vi "execute_value_write_policy.vi"(8 "error in (no error)":errorcluster, 9 "Publish Time":timestamp, 10 "New Topic Value":variant, 11 "BasicSubscription In":refnum<class "BasicSubscription.lvclass">) -> (0 "error out":errorcluster, 3 "BasicSubscription Out":refnum<class "BasicSubscription.lvclass">)   [LabVIEW 2015, in "SubscriptionPolicy.lvlib" / "BasicSubscription.lvclass"]
uses:
  BasicSubscription.lvclass
  IMediator/ISubscriptionPolicy/ISubscriptionPolicy.lvclass/ISubscriptionPolicy.ctl
  IMediator/ITransport/ITransport.lvclass
  IMediator/ISubscriptionPolicy/ISubscriptionPolicy.lvclass
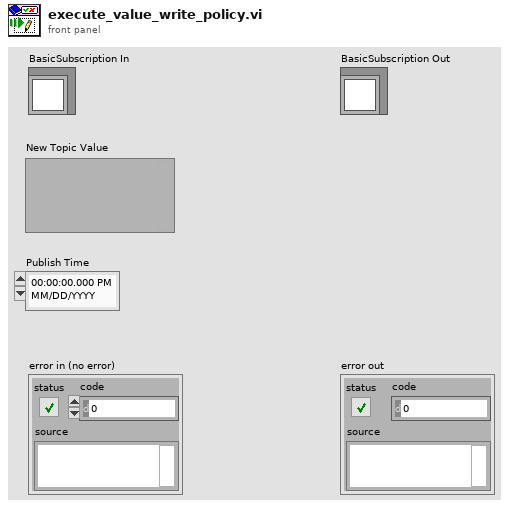
[diagram p1: front panel]
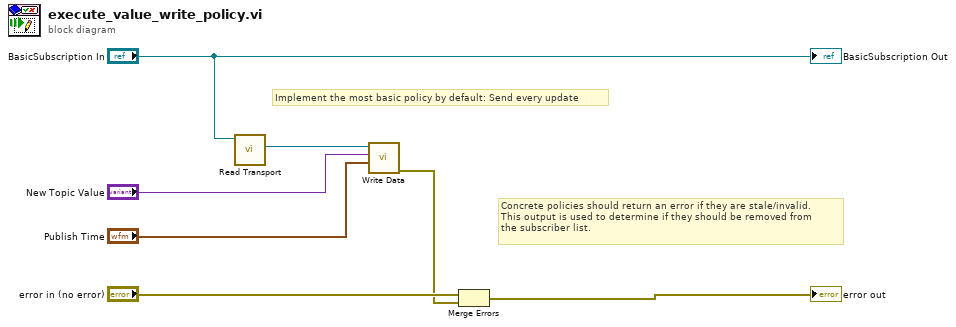
[diagram p0: block diagram]
diagram:
  # "Implement the most basic policy by default: Send every update"
  # "Concrete policies should return an error if they are stale/invalid.\nThis output is used to determine if they should be removed from\nthe subscriber list."
  n1 = call "Read Transport.vi"("ISubscriptionPolicy in"="BasicSubscription In") -> ("Transport"=w6:refnum<class "ITransport.lvclass">)  [unwired: 10 in]
  n2 = call-dynamic "Write Data.vi"("Publication Time"="Publish Time", "Value"="New Topic Value", "ITransport in"=w6) -> ("error out"=w2:errorcluster)  [unwired: 7 in, 1 out]
  n3 = Merge Errors("error in (no error)", w2) -> (→"error out":errorcluster)
  "BasicSubscription Out" <- "BasicSubscription In"
